vi "Get Channel Info.vi"(6 "Device Ref in":T1 format="%.0x", 7 "Command?":bool, 8 "error in (no error)":errorcluster, 9 "Item GUID":string, 10 "Channel Refs in":T2 {"Trigger Data Refs"."Data Reference" format="%.0x"; "Trigger Chan Refs" format="%.0x"; "System Time"."Get Date-Time Channel Data Ref" format="%.0x"; "System Time"."Absolute Time Channel Data Ref" format="%.0x"; "System Time"."Channel Data Reference" format="%.0x"; "Status Data Refs"."Data Reference" format="%.0x"; "Command Data Refs"."Data Reference" format="%.0x"; "Status Chan Refs" format="%.0x"; "Command Chan Refs" format="%.0x"}, 11 "Item Ref in":T1 format="%.0x") -> (0 "error out":errorcluster, 1 "Channel out":T6 {"Data Ref" format="%.0x"}, 2 "Channel Refs out":T2 {"Trigger Data Refs"."Data Reference" format="%.0x"; "Trigger Chan Refs" format="%.0x"; "System Time"."Get Date-Time Channel Data Ref" format="%.0x"; "System Time"."Absolute Time Channel Data Ref" format="%.0x"; "System Time"."Channel Data Reference" format="%.0x"; "Status Data Refs"."Data Reference" format="%.0x"; "Command Data Refs"."Data Reference" format="%.0x"; "Status Chan Refs" format="%.0x"; "Command Chan Refs" format="%.0x"}, 3 "Item Ref out":T1 format="%.0x")   [LabVIEW 2012, in "Waveform Data Logger Engine.lvlib"]
uses:
  Waveform Data Logger Engine.lvlib
  Types/Channel.ctl
  <vilib>/NI Veristand/Custom Device API/Data Reference.ctl
  Types/Channels.ctl
  <vilib>/NI Veristand/Custom Device API/Custom Device Item Ref.ctl
  <vilib>/NI Veristand/Custom Device API/Block Data Reference.ctl
  Types/System Time.ctl
  <vilib>/NI Veristand/Custom Device API/Data Access Type.ctl
  <vilib>/NI Veristand/Custom Device Tools/Custom Device Utility Library/NI VeriStand - Search for Item by GUID.vi
  <vilib>/NI VeriStand/Custom Device Tools/Custom Device Utility Library/Custom Device Utility Library.lvlib
  <vilib>/NI VeriStand/Custom Device API/Custom Device API.lvlib
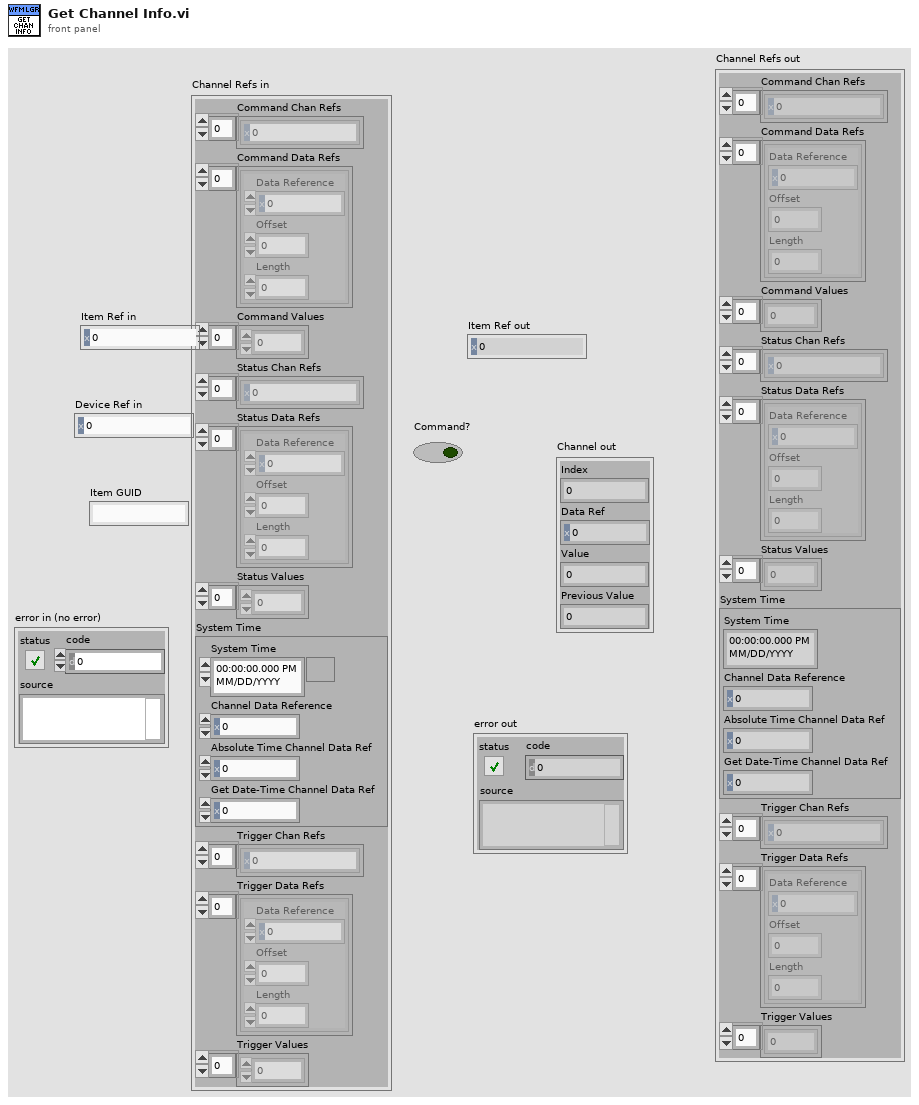
[diagram p1: front panel]
types:
  T1 = typedef "Custom Device API.lvlib/Custom Device Item Ref.ctl" = u64
  T2 = typedef "Waveform Data Logger Engine.lvlib/Channels.ctl" = cluster{"Command Chan Refs":T1[], "Command Data Refs":T3[], "Command Values":dbl[], "Status Chan Refs":T1[], "Status Data Refs":T3[], "Status Values":dbl[], "System Time":T5, "Trigger Chan Refs":T1[], "Trigger Data Refs":T3[], "Trigger Values":dbl[]}
  T3 = typedef "Custom Device API.lvlib/Block Data Reference.ctl" = cluster{"Data Reference":T4, "Offset":i32, "Length":i32}
  T4 = typedef "Custom Device API.lvlib/Data Reference.ctl" = i32
  T5 = typedef "Waveform Data Logger Engine.lvlib/System Time.ctl" = cluster{"System Time":timestamp, "Data Reference":T4, "Absolute Time Channel Data Ref":T4, "Get Date-Time Channel Data Ref":T4}
  T6 = typedef "Waveform Data Logger Engine.lvlib/Channel.ctl" = cluster{"Index":i32, "Data Ref":T4, "Value":dbl, "Previous Value":dbl}
  T7 = typedef "Custom Device API.lvlib/Data Access Type.ctl" = enum16{"Read", "Write"}
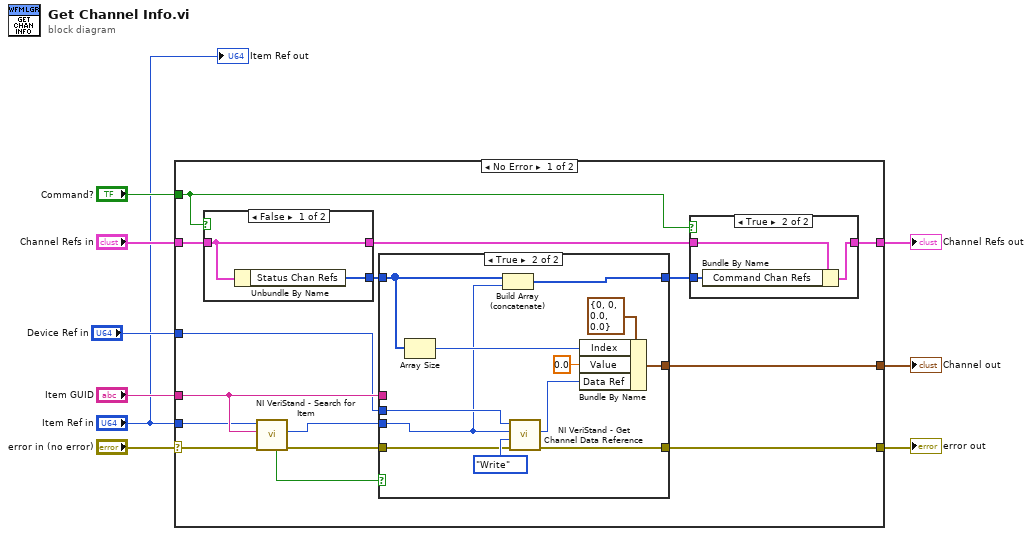
[diagram p0: block diagram]
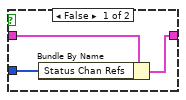
[diagram p3: hidden frame]
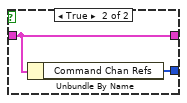
[diagram p4: hidden frame]
diagram:
  n1 = case shown="No Error" "error in (no error)" {
    selector: "error in (no error)" -> [w21 w49]
    tunnel: "Channel Refs in" -> [w24 w50]
    tunnel: "Command?" -> [w14 _]
    tunnel: [w22 w50] -> w6
    tunnel: [w20 w49] -> w5
    tunnel: [w15 _] -> w4
    tunnel: "Item GUID" -> [w12 _]
    tunnel: "Item Ref in" -> [w11 _]
    tunnel: "Device Ref in" -> [w10 _]
    frame No Error {
      n2 = case shown="False" w14 {
        tunnel: w24 -> [w46 w48]
        tunnel: [w46 w48] -> w23
        tunnel: [w45 w47] -> w19
        frame False {
          n3 = Unbundle By Name(w46) -> ("Status Chan Refs"=w45:T1[])
        }
        frame True {
          n4 = Unbundle By Name(w48) -> ("Command Chan Refs"=w47:T1[])
        }
      }
      n5 = call-poly <vilib>:"NI VeriStand - Search for Item.vi"("error in"=w21, "Item GUID"=w12, "Section Ref in"=w11) -> ("error out"=w17:errorcluster, "Item Ref"=w16:T1, "Found"=w13:bool)  [unwired: 6 out]
      n6 = case shown="True" w13 {
        tunnel: w10 -> [_ w37]
        tunnel: [w26 w35] -> w20
        tunnel: w19 -> [w25 w33]
        tunnel: [w25 w32] -> w18
        tunnel: w17 -> [w26 w31]
        tunnel: w16 -> [_ w29]
        tunnel: [_ w30] -> w15
        tunnel: w12 -> [_ _]
        frame False {
        }
        frame True {
          n7 = Array Size(array=w33) -> (size(s)=w34:i32)
          n8 = Build Array (concatenate)(w33, w29) -> (w32:T1[])
          n9 = call <vilib>:"NI VeriStand - Get Channel Data Reference.vi"("error in (no error)"=w31, "Access"=Data_Access_Type."Write", "Channel Ref in"=w29, "Device Ref in"=w37) -> ("error out"=w35:errorcluster, "Channel Data Reference"=w28:T4)  [unwired: 5 in, 1 out]
          n10 = Bundle By Name(cluster=T6 {"Index"=0, "Data Ref"=0, "Value"=0.0, "Previous Value"=0.0} ("Channel out"), "Index"=w34, "Value"=0.0, "Data Ref"=w28) -> (w30:T6)
        }
      }
      n11 = case shown="True" w14 {
        tunnel: w23 -> [w41 w44]
        tunnel: [w40 w43] -> w22
        tunnel: w18 -> [w39 w42]
        frame False {
          n12 = Bundle By Name(cluster=w41, "Status Chan Refs"=w39) -> (w40:T2)
        }
        frame True {
          n13 = Bundle By Name(cluster=w44, "Command Chan Refs"=w42) -> (w43:T2)
        }
      }
    }
    frame Error {
    }
  }
  "error out" <- w5
  "Channel out" <- w4
  "Channel Refs out" <- w6
  "Item Ref out" <- "Item Ref in"
